vi "Connect.vi"(0 "reference in":refnum<class "Database_ODBC.lvclass">, 11 "error in (no error)":errorcluster) -> (4 "reference out":refnum<class "Database_ODBC.lvclass">, 15 "error out":errorcluster)   [LabVIEW 2019, in "Database_ODBC.lvclass"]
uses:
  Database_ODBC.lvclass
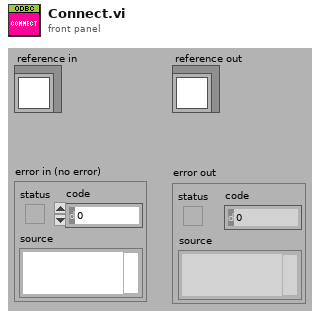
[diagram p1: front panel]
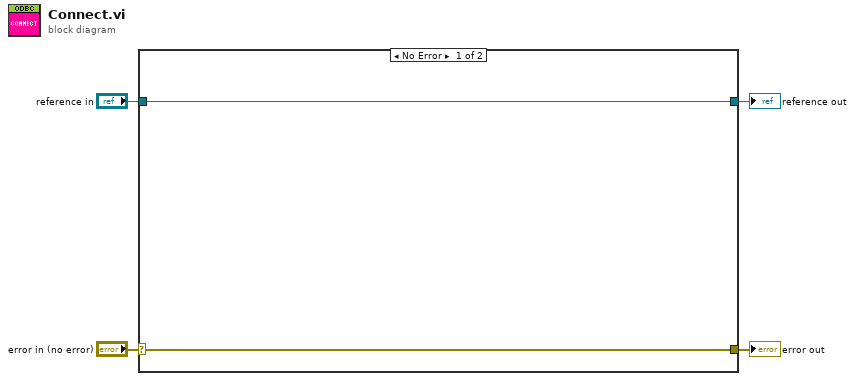
[diagram p0: block diagram]
diagram:
  n1 = case shown="No Error" "error in (no error)" {
    selector: "error in (no error)" -> [w6 w8]
    tunnel: [w6 w8] -> w3
    tunnel: [w5 w7] -> w1
    tunnel: "reference in" -> [w5 w7]
    frame No Error {
    }
    frame Error {
    }
  }
  "error out" <- w3
  "reference out" <- w1
